vi "Teleop.vi"(10 "Match Info":T1={"Autonomous Elapsed Seconds"=0.0, "TeleOp Elapsed Seconds"=0.0, "Disabled Elapsed Seconds"=0.0, "Visited Autonomous"=FALSE, "Visited TeleOp"=FALSE, "Visited Disabled"=FALSE, "Autonomous Settings"={"Autonomous Style"=enum."Independent", "VI Refnum"=refnum}}, 11 "Call Context":T2) -> ()   [LabVIEW 2016]
doc: "This VI is called for each TeleOp packet received from the DS where the robot is not disabled. It is often used to read from the joysticks and update I/O or to update setpoints for timed control loops. It should complete and return within 20 milliseconds or it may miss DS packets."
uses:
  <vilib>/Rock Robotics/Network Tables/NT Write Numeric Array.vi
  <vilib>/Rock Robotics/Network Tables/NT Read Boolean.vi
  Encoder Rate.vi
  <vilib>/Rock Robotics/WPI/RobotDrive/WPI_RobotDriveMecanumDrive_Cartesian.vi
  <vilib>/Rock Robotics/Network Tables/NT Write Boolean Array.vi
  <vilib>/Rock Robotics/Network Tables/NT Read Number.vi
  <vilib>/Rock Robotics/WPI/DriverStation/WPI_DriverStationMatch Info.ctl
  <vilib>/Rock Robotics/WPI/DriverStation/WPI_DriverStationDerivedRobotMode.ctl
panel:
  out "Type 2":bool
  out "Type 1":bool
  in  "Spin Control":dbl
  in  "Minimum 2":dbl
  in  "Maximum 2":dbl
  in  "Shooter Control":dbl=0.5
  out "Boolean":bool
  out "Sample Slider 0":dbl(slide) scale=0.0..5.0
  out "Sample Boolean 1":bool
  out "Sample Boolean 0":bool
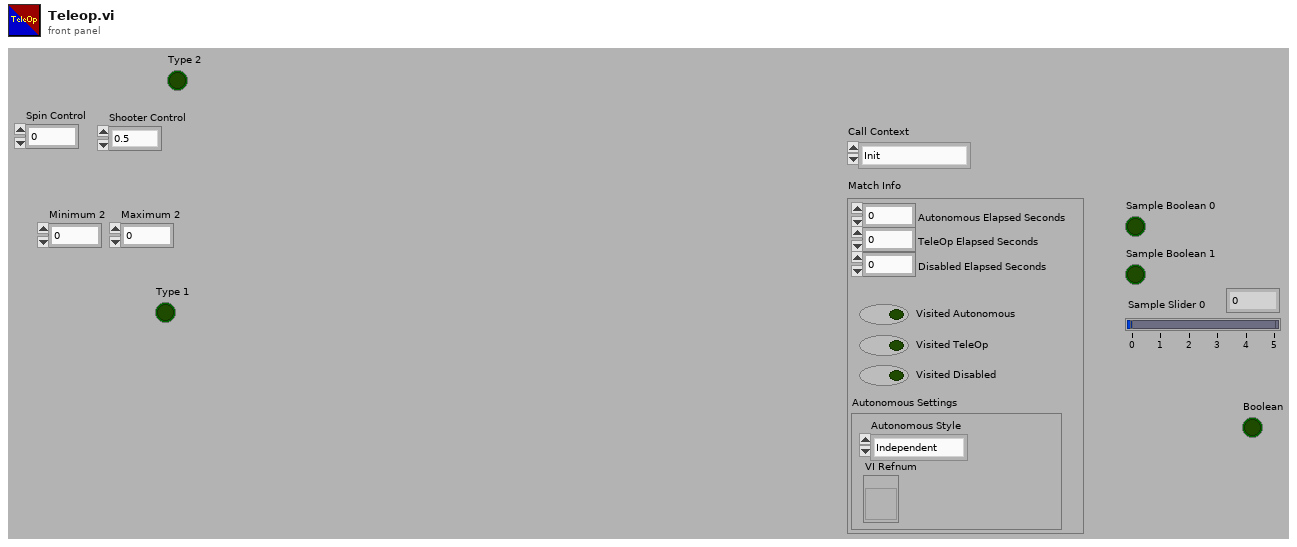
[diagram p1: front panel]
types:
  T1 = typedef "WPI_DriverStationMatch Info.ctl" = cluster{"Autonomous Elapsed Seconds":dbl, "TeleOp Elapsed Seconds":dbl, "Disabled Elapsed Seconds":dbl, "Visited Autonomous":bool, "Visited TeleOp":bool, "Visited Disabled":bool, "Autonomous Settings":cluster{"Autonomous Style":enum16{"Iterative", "Independent"}, "VI Refnum":refnum<vi>}}
  T2 = typedef "WPI_DriverStationDerivedRobotMode.ctl" = enum16{"Init", "Execute", "Stop"}
  T3 = typedef "WPI_RobotDriveDevRef.ctl" = cluster{"DevStatus":errorcluster, "Motors[]":T4[], "Square Inputs":bool, "Max Output":dbl}
  T4 = typedef "WPI_MotorControlDeviceRef.ctl" = cluster{"DeviceStatus":errorcluster, "Type":T5, "PWM":cluster{"PWM Channel":T6, "DeadBand":T7}, "CAN":cluster{"Device Number":u8, "SetOutput VI Ref":variant, "GetOutput VI Ref":variant, "Enable VI Ref":variant, "Disable VI Ref":variant, "Data":variant}, "Invert":bool}
  T5 = typedef "WPI_MotorControlType.ctl" = enum16{"PWM", "CAN"}
  T6 = typedef "FPGA_DIOPWMChannel.ctl" = enum8{"PWM 0", "PWM 1", "PWM 2", "PWM 3", "PWM 4", "PWM 5", "PWM 6", "PWM 7", "PWM 8", "PWM 9", "PWM MXP 0", "PWM MXP 1", "PWM MXP 2", "PWM MXP 3", "PWM MXP 4", "PWM MXP 5", "PWM MXP 6", "PWM MXP 7", "PWM MXP 8", "PWM MXP 9", "Invalid"}
  T7 = typedef "WPI_PWMDeadband.ctl" = cluster{"Name":string, "maxPositivePwm":i32, "minPositivePwm":i32, "centerPwm":i32, "maxNegativePwm":i32, "minNegativePwm":i32, "angularRange":u16}
  T8 = typedef "WPI_JoystickDevRef.ctl" = cluster{"Device":T9}
  T9 = typedef "WPI_JoystickDeviceEnum.ctl" = enum16{"USB 0", "USB 1", "USB 2", "USB 3", "USB 4", "USB 5"}
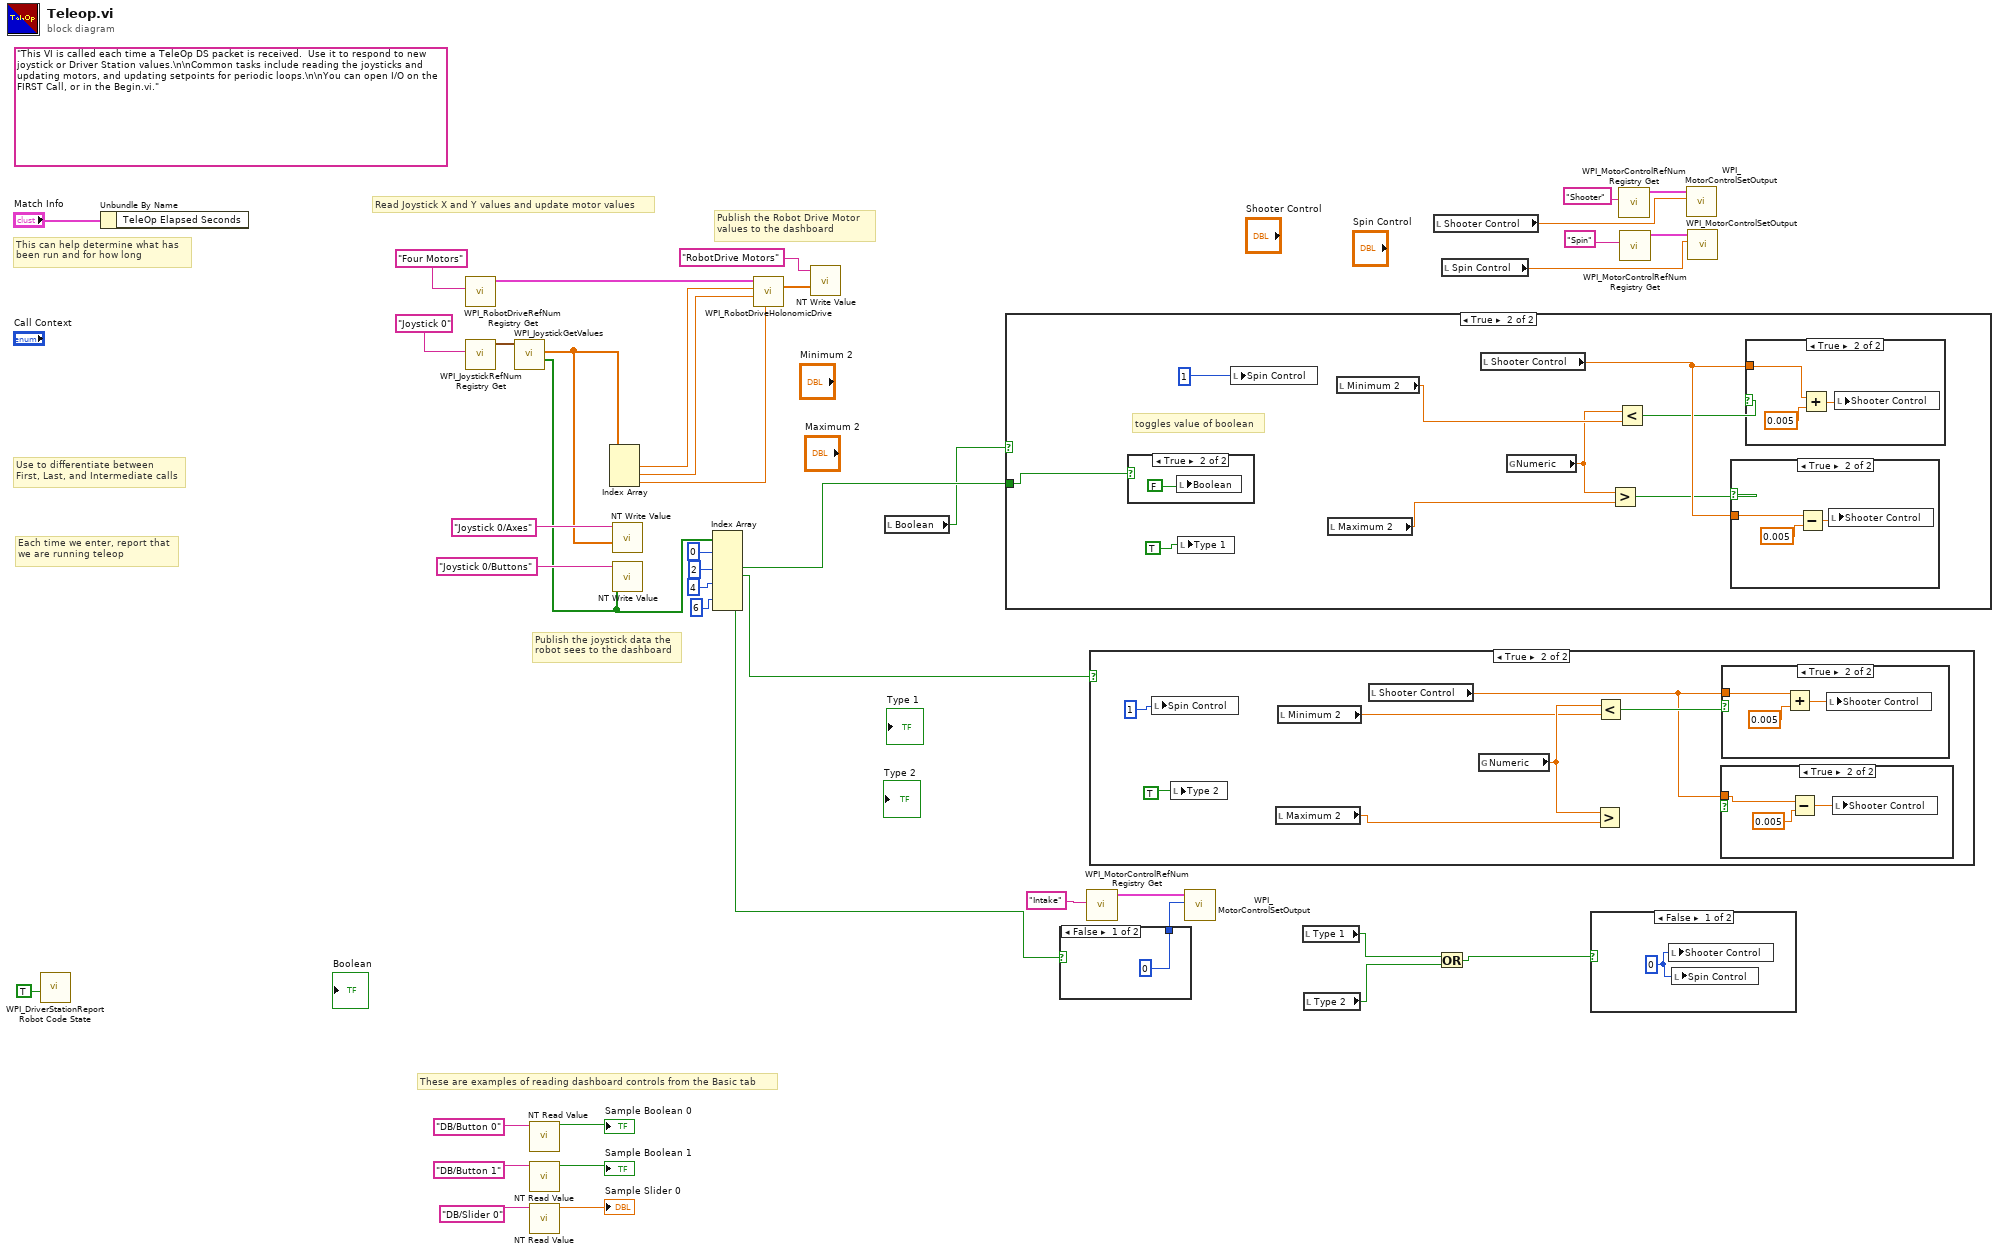
[diagram p0: block diagram]
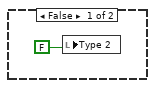
[diagram p3: hidden frame]
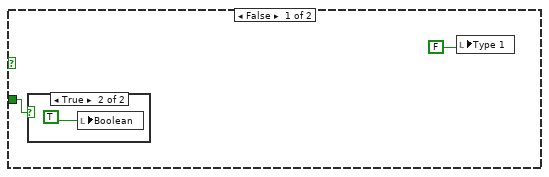
[diagram p6: hidden frame]
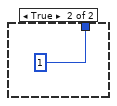
[diagram p11: hidden frame]
diagram:
  (unwired) "This VI is called each time a TeleOp DS packet is received.  Use it to respond to new joystick or Driver Station values.\n\nCommon tasks include reading the joysticks and updating motors, and updating setpoints for periodic loops.\n\nYou can open I/O on the FIRST Call, or in the Begin.vi."
  # "These are examples of reading dashboard controls from the Basic tab"
  # "Publish the Robot Drive Motor\nvalues to the dashboard"
  # "Publish the joystick data the\nrobot sees to the dashboard"
  # "Each time we enter, report that\nwe are running teleop"
  # "Use to differentiate between\nFirst, Last, and Intermediate calls"
  # "This can help determine what has\nbeen run and for how long"
  # "Read Joystick X and Y values and update motor values"
  n1 = call <vilib>:"WPI_DriverStationReport Robot Code State.vi"("TeleOp"=TRUE ("Autonomous")) -> ()  [unwired: 10 in, 1 out]
  n2 = Unbundle By Name("Match Info") -> ()  [unwired: 1 out]
  n3 = call <vilib>:"WPI_RobotDriveRefNum Registry Get.vi"("refnum name"="Four Motors") -> ("RobotDriveDevRef"=w39:T3)  [unwired: 1 in, 9 out]
  n4 = call <vilib>:"WPI_JoystickRefNum Registry Get.vi"("refnum name"="Joystick 0") -> ("JoystickDevRef"=w36:T8)  [unwired: 1 in, 9 out]
  n5 = call <vilib>:"WPI_JoystickGetValues.vi"("JoystickDevRef"=w36) -> ("Buttons"=w4:bool[], "Axes"=w31:dbl[])  [unwired: 6 in, 3 out]
  n6 = call-poly <vilib>:"NT Read Value.vi"("Name"="DB/Button 0" ("refnum name")) -> ("Boolean"=→"Sample Boolean 0":bool)  [unwired: 9 in, 1 out]
  n7 = call-poly <vilib>:"NT Read Value.vi"("Name"="DB/Button 1" ("refnum name")) -> ("Boolean"=→"Sample Boolean 1":bool)  [unwired: 9 in, 1 out]
  n8 = call-poly <vilib>:"NT Read Value.vi"("Name"="DB/Slider 0" ("refnum name")) -> ("Numeric"=→"Sample Slider 0":dbl)  [unwired: 9 in, 1 out]
  n9 = Index Array(array=w31) -> (element #1=w38:dbl, element #2=w33:dbl, element #3=w34:dbl)  [unwired: 3 in]
  n10 = call-poly <vilib>:"NT Write Value.vi"("Numeric Array"=w31, "Name"="Joystick 0/Axes") -> ()  [unwired: 9 in, 1 out]
  n11 = call-poly <vilib>:"NT Write Value.vi"("Boolean Array"=w4, "Name"="Joystick 0/Buttons") -> ()  [unwired: 9 in, 1 out]
  n12 = Index Array(array=w4, index #1=0, index #3=2, index #5=4, index #7=6) -> (element #3=w15:bool, element #4=w5:bool, element #7=w16:bool)  [unwired: 4 in, 5 out]
  n13 = call-poly <vilib>:"WPI_RobotDriveHolonomicDrive.vi"("Rotation"=w34, "Y"=w33, "X"=w38, "RobotDriveDevRef"=w39) -> ("Motor Values"=w29:dbl[])  [unwired: 5 in, 2 out]
  n14 = call-poly <vilib>:"NT Write Value.vi"("Numeric Array"=w29, "Name"="RobotDrive Motors") -> ()  [unwired: 9 in, 1 out]
  n15 = local read "Boolean"() -> (w6:bool)
  n16 = case shown="True" w6 {
    tunnel: w15 -> [w43 w46]
    frame False {
      n17 = case shown="True" w43 {
        frame False {
        }
        frame True {
          n18 = local write "Boolean"(TRUE) -> ()
        }
      }
      n19 = local write "Type 1"(FALSE) -> ()
    }
    frame True {
      # "toggles value of boolean"
      n20 = case shown="True" w46 {
        frame False {
        }
        frame True {
          n21 = local write "Boolean"(FALSE) -> ()
        }
      }
      n22 = local write "Type 1"(TRUE) -> ()
      n23 = local write "Spin Control"(1) -> ()
      n24 = local read "Maximum 2"() -> (w52:dbl)
      n25 = local read "Minimum 2"() -> (w51:dbl)
      n26 = local read "Shooter Control"() -> (w53:dbl)
      n27 = global read "Encoder Rate.vi" "Numeric"() -> (w48:dbl)
      n28 = Greater?(x=w48, y=w52) -> (0:w50:bool)
      n29 = Less?(x=w48, y=w51) -> (x < y?=w49:bool)
      n30 = case shown="True" w50 {
        tunnel: w53 -> [_ w55]
        frame False {
        }
        frame True {
          n31 = Subtract(x=w55, y=0.005) -> (x-y=w56:dbl)
          n32 = local write "Shooter Control"(w56) -> ()
        }
      }
      n33 = case shown="True" w49 {
        tunnel: w53 -> [_ w58]
        frame False {
        }
        frame True {
          n34 = Add(x=w58, y=0.005) -> (x+y=w59:dbl)
          n35 = local write "Shooter Control"(w59) -> ()
        }
      }
    }
  }
  n36 = case shown="False" w16 {
    tunnel: [0 1] -> w18
    frame False {
    }
    frame True {
    }
  }
  n37 = call <vilib>:"WPI_MotorControlRefNum Registry Get.vi"("refnum name"="Intake") -> ("MotorControlDevRef"=w21:T4)  [unwired: 9 in, 1 out]
  n38 = case shown="True" w5 {
    frame False {
      n39 = local write "Type 2"(FALSE) -> ()
    }
    frame True {
      n40 = local write "Spin Control"(1) -> ()
      n41 = local write "Type 2"(TRUE) -> ()
      n42 = local read "Maximum 2"() -> (w69:dbl)
      n43 = local read "Minimum 2"() -> (w68:dbl)
      n44 = local read "Shooter Control"() -> (w65:dbl)
      n45 = global read "Encoder Rate.vi" "Numeric"() -> (w70:dbl)
      n46 = Greater?(x=w70, y=w69) -> ()  [unwired: 1 out]
      n47 = Less?(x=w70, y=w68) -> (x < y?=w66:bool)
      n48 = case shown="True" {
        selector: _ -> [_ _]
        tunnel: w65 -> [_ w72]
        frame False {
        }
        frame True {
          n49 = Subtract(x=w72, y=0.005) -> (x-y=w71:dbl)
          n50 = local write "Shooter Control"(w71) -> ()
        }
      }
      n51 = case shown="True" w66 {
        tunnel: w65 -> [_ w75]
        frame False {
        }
        frame True {
          n52 = Add(x=w75, y=0.005) -> (x+y=w74:dbl)
          n53 = local write "Shooter Control"(w74) -> ()
        }
      }
    }
  }
  n54 = call <vilib>:"WPI_MotorControlSetOutput.vi"("Output"=w18, "MotorControlDevRef"=w21) -> ()  [unwired: 7 in, 3 out]
  n55 = local read "Type 1"() -> (w3:bool)
  n56 = local read "Type 2"() -> (w2:bool)
  n57 = local read "Shooter Control"() -> (w10:dbl)
  n58 = Or(x=w3, y=w2) -> (x .or. y?=w1:bool)
  n59 = local read "Spin Control"() -> (w9:dbl)
  n60 = case shown="False" w1 {
    frame False {
      w77 = 0
      n61 = local write "Shooter Control"(w77) -> ()
      n62 = local write "Spin Control"(w77) -> ()
    }
    frame True {
    }
  }
  n63 = call <vilib>:"WPI_MotorControlRefNum Registry Get.vi"("refnum name"="Shooter") -> ("MotorControlDevRef"=w12:T4)  [unwired: 9 in, 1 out]
  n64 = call <vilib>:"WPI_MotorControlRefNum Registry Get.vi"("refnum name"="Spin") -> ("MotorControlDevRef"=w14:T4)  [unwired: 9 in, 1 out]
  n65 = call <vilib>:"WPI_MotorControlSetOutput.vi"("Output"=w10, "MotorControlDevRef"=w12) -> ()  [unwired: 7 in, 3 out]
  n66 = call <vilib>:"WPI_MotorControlSetOutput.vi"("Output"=w9, "MotorControlDevRef"=w14) -> ()  [unwired: 7 in, 3 out]
